vi "MFC 10Hz.vi"() -> ()   [LabVIEW 2014]
uses:
  <vilib>/rvi/Emulation/niFpgaGetClockAttributes.vi
  <vilib>/rvi/Emulation/niFpgaSctlEmulationGetInTimedLoop.vi
  <vilib>/rvi/Emulation/niFpgaEmulationReportErrorSimple.vi
  <vilib>/rvi/Emulation/niFpgaCriticalErrorInLSC.vi
panel:
  in  "Count(mSec)":u32=100
  out "MFC CO-1 out":u8[](array[numeric])
  out "MFC HC-1 out":u8[](array[numeric])
  out "MFC AIR-1 out":u8[](array[numeric])
  out "MFC NO-1 out":u8[](array[numeric])
  out "MFC Air-B out":u8[](array[numeric])
  in  "MFC OUT Array":u8[](array[numeric])=[66, 48, 48, 48, 48, 48, 13, 67, 48, 48, 48, 48, 48, 13, 73, 48, 48, 48, 48, 48, 13, 74, 48, 48, 48, 48, 48, 13, 75, 48, 48, 48, 48, 48, 13, 76, 48, 48, 48, 48, 48, 13, 0, 0, 0, 0, 0, 0, 0, 0, 0, 0, 0, 0, 0, 0]
  out "MFC IN Array":u8[](array[numeric])
  out "MFC HC-B out":u8[](array[numeric])
  out "MFC Air-2 out":u8[](array[numeric])
  out "MFC HC-2 out":u8[](array[numeric])
  out "MFC error No.":u8
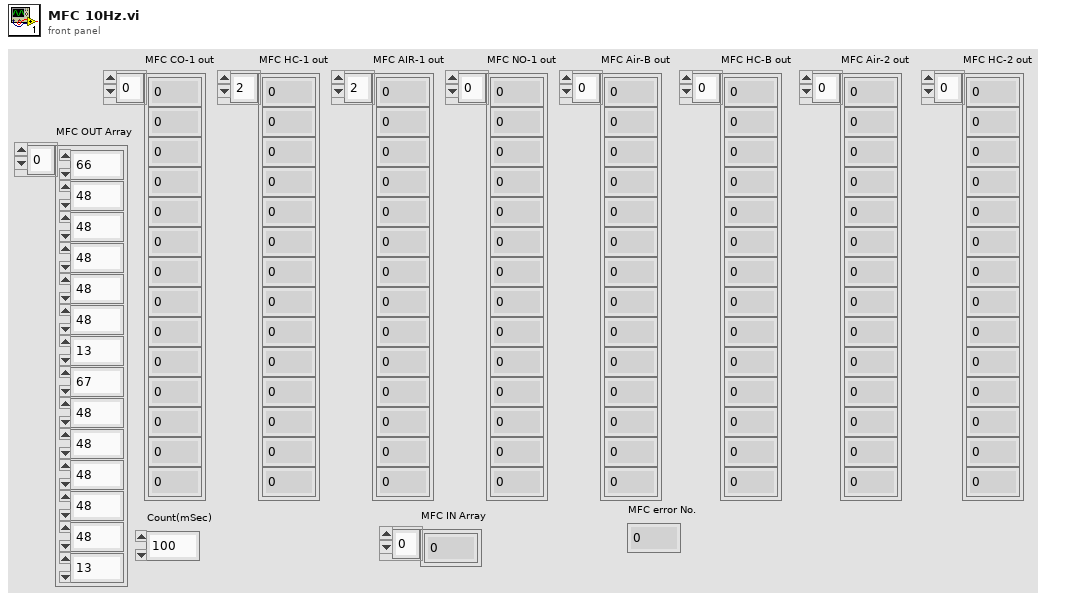
[diagram p1: front panel]
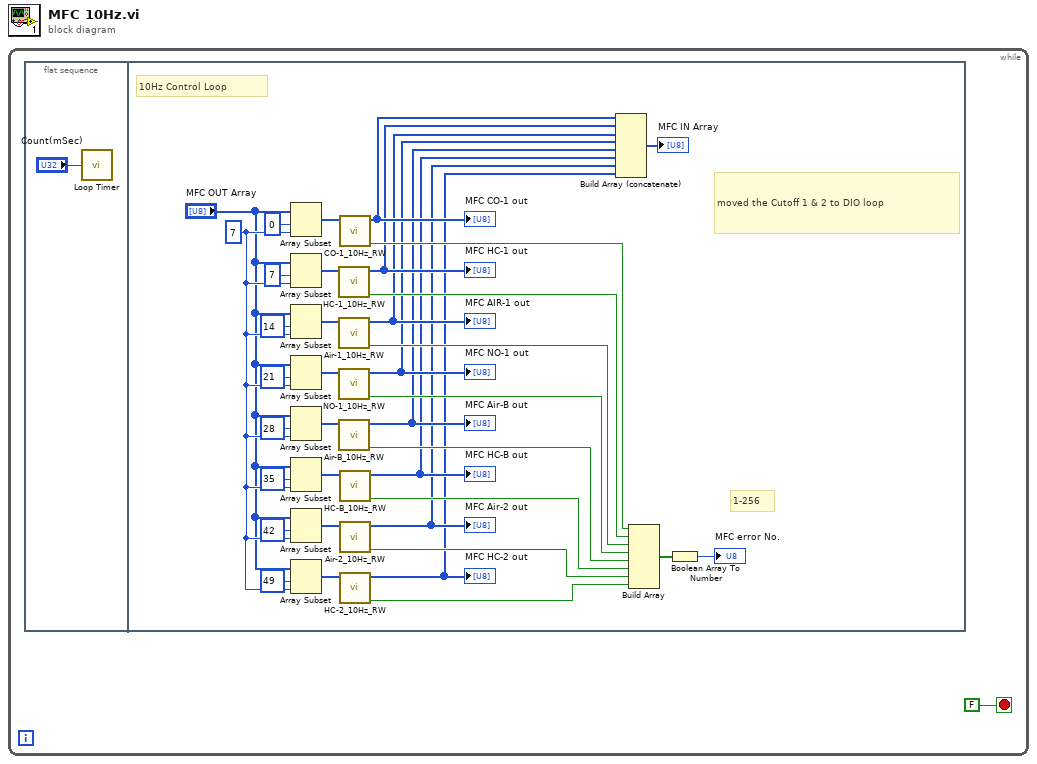
[diagram p0: block diagram]
diagram:
  n1 = while {
    stop <- FALSE stop-if-true
    n2 = flat-sequence {
      frame #0 {
        n3 = call "Loop Timer"("Count(mSec)"="Count(mSec)") -> ()  [unwired: 1 out]
      }
      frame #1 {
        w31 = 7 ("length")
        # "1-256"
        # "10Hz Control Loop"
        # "moved the Cutoff 1 & 2 to DIO loop"
        n4 = Array Subset(array="MFC OUT Array", index=0, length=w31) -> (w26:u8[])
        n5 = Array Subset(array="MFC OUT Array", index=7, length=w31) -> (w23:u8[])
        n6 = Array Subset(array="MFC OUT Array", index=14, length=w31) -> (w21:u8[])
        n7 = Array Subset(array="MFC OUT Array", index=21, length=w31) -> (w19:u8[])
        n8 = Array Subset(array="MFC OUT Array", index=28, length=w31) -> (w17:u8[])
        n9 = Array Subset(array="MFC OUT Array", index=35, length=w31) -> (w16:u8[])
        n10 = Array Subset(array="MFC OUT Array", index=42, length=w31) -> (w14:u8[])
        n11 = Array Subset(array="MFC OUT Array", index=49, length=w31) -> (w12:u8[])
        n12 = call "HC-1_10Hz_RW.vi"("Byte Array"=w23) -> ("Fault"=w22:bool, "MFC out"=w10:u8[])  [unwired: 9 in]
        "MFC HC-1 out" <- w10
        n13 = call "Air-1_10Hz_RW.vi"("Byte Array"=w21) -> ("Fault"=w20:bool, "MFC out"=w9:u8[])  [unwired: 9 in]
        "MFC AIR-1 out" <- w9
        n14 = call "NO-1_10Hz_RW.vi"("Byte Array"=w19) -> ("Fault"=w18:bool, "MFC out"=w8:u8[])  [unwired: 9 in]
        "MFC NO-1 out" <- w8
        n15 = call "Air-B_10Hz_RW.vi"("Byte Array"=w17) -> ("Fault"=w6:bool, "MFC out"=w7:u8[])  [unwired: 9 in]
        "MFC Air-B out" <- w7
        n16 = call "CO-1_10Hz_RW.vi"("Byte Array"=w26) -> ("Fault"=w24:bool, "MFC out"=w25:u8[])  [unwired: 9 in]
        "MFC CO-1 out" <- w25
        n17 = call "HC-B_10Hz_RW.vi"("Byte Array"=w16) -> ("Fault"=w15:bool, "MFC out"=w5:u8[])  [unwired: 9 in]
        "MFC HC-B out" <- w5
        n18 = call "Air-2_10Hz_RW.vi"("Byte Array"=w14) -> ("Fault"=w13:bool, "MFC out"=w4:u8[])  [unwired: 9 in]
        "MFC Air-2 out" <- w4
        n19 = call "HC-2_10Hz_RW.vi"("Byte Array"=w12) -> ("Fault"=w11:bool, "MFC out"=w3:u8[])  [unwired: 9 in]
        "MFC HC-2 out" <- w3
        n20 = Build Array (concatenate)(w25, w10, w9, w8, w7, w5, w4, w3) -> (→"MFC IN Array":u8[])
        n21 = Build Array(w24, w22, w20, w18, w6, w15, w13, w11) -> (w29:bool[])
        n22 = Boolean Array To Number(Boolean array=w29) -> (number=→"MFC error No.":u8)
      }
    }
  }
